vi "LV to ITX 2.2 2D w X&Y.vi"(0 "Commands":string, 1 "Kill X&Y waves?":bool=TRUE, 4 "Y Array name":string, 5 "filename":path, 6 "Y 1D Array":dbl[](array[numeric]), 7 "Notes":string, 8 "X  Array name":string, 9 "X 1D Array":dbl[](array[numeric]), 10 "2D Array name":string, 11 "2D Array":dbl[][](array[numeric])) -> (3 "file":path)   [LabVIEW 2016, in "LV to ITX.lvclass"]
uses:
  LV to ITX.lvclass
panel:
  out "Commands":string
  out "String":string
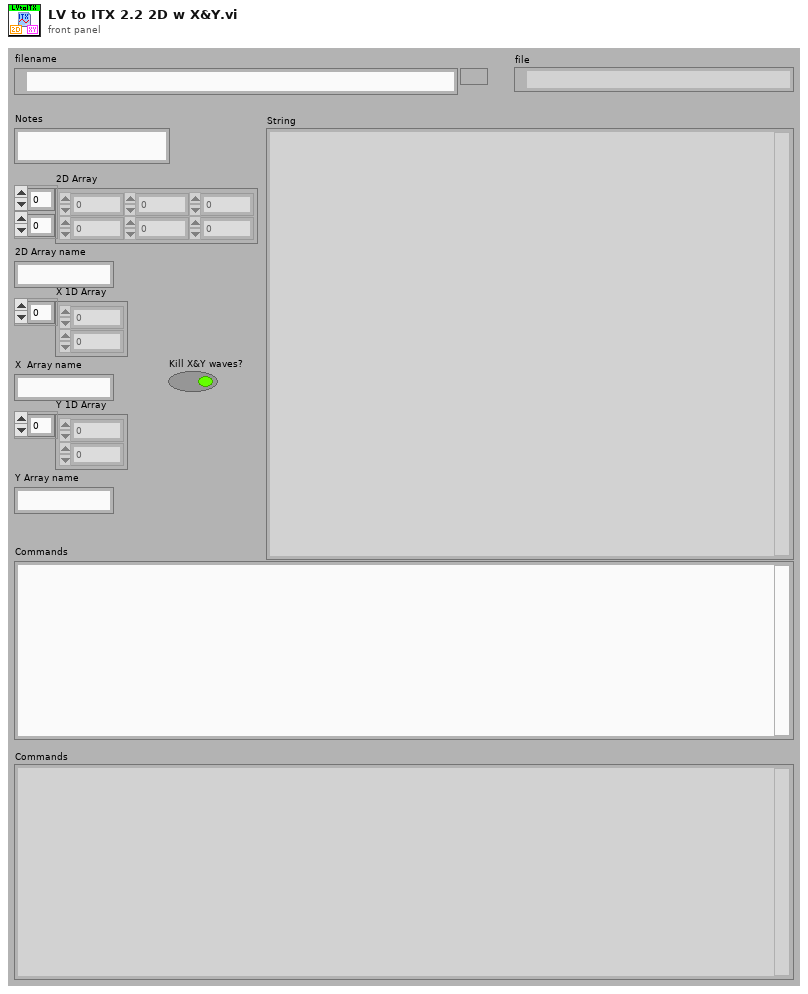
[diagram p1: front panel]
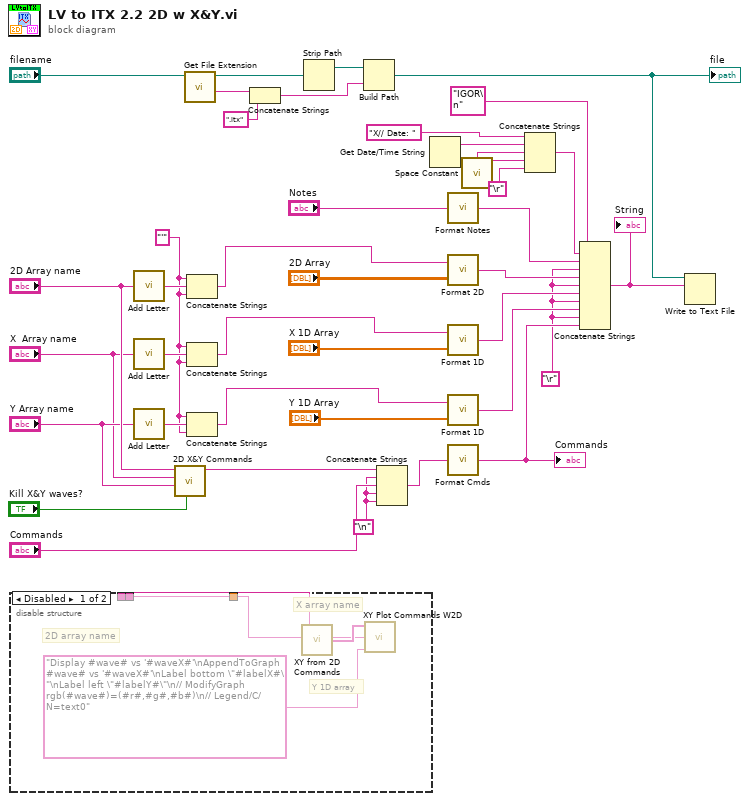
[diagram p0: block diagram]
diagram:
  w13 = "'" ("string")
  w2 = "\n"
  w27 = "\r"
  n1 = disable-structure shown="Disabled" {
    disable-tunnel: _ -> [w45 _]
    disable-tunnel: _ -> [w44 _]
    disable-tunnel: _ -> [w41 _]
    frame Disabled {
      # "Y 1D array"
      # "2D array name"
      # "X array name"
      n2 = call "XY from 2D Commands.vi"("Y 1D Array"=w44, "2D wave"=w45) -> ("wavenames"=w43:string[])
      n3 = call "XY Plot Commands W2D.vi"("wavenames"=w43, "input string"="Display #wave# vs '#waveX#'\nAppendToGraph #wave# vs '#waveX#'\nLabel bottom \"#labelX#\"\nLabel left \"#labelY#\"\n// ModifyGraph rgb(#wave#)=(#r#,#g#,#b#)\n// Legend/C/N=text0", "X wave"=w41) -> ()  [unwired: 2 in, 1 out]
    }
    frame Enabled {
    }
  }
  n4 = call "Add Letter.vi"("String"="2D Array name") -> ("output string"=w16:string)
  n5 = call "Add Letter.vi"("String"="X  Array name") -> ("output string"=w15:string)
  n6 = call "Add Letter.vi"("String"="Y Array name") -> ("output string"=w14:string)
  n7 = call "2D X&Y Commands.vi"("Kill X&Y waves?"="Kill X&Y waves?", "Y wave"="Y Array name", "X wave"="X  Array name", "2D wave"="2D Array name") -> ("result string"=w7:string)  [unwired: 6 in, 1 out]
  n8 = call <vilib>:"Get File Extension.vi"("file"="filename") -> ("filename without extension"=w23:string, "dup file"=w20:path)  [unwired: 1 in, 8 out]
  n9 = Concatenate Strings(w13, w16, w13) -> (w10:string)
  n10 = Concatenate Strings(w13, w15, w13) -> (w11:string)
  n11 = Concatenate Strings(w13, w14, w13) -> (w12:string)
  n12 = Concatenate Strings(w23, ".itx") -> (w18:string)
  n13 = Strip Path(path=w20) -> (stripped path=w19:path)  [unwired: 1 out]
  n14 = Build Path(base path=w19, name or relative path=w18) -> (appended path=w3:path)
  "file" <- w3
  n15 = Concatenate Strings(w7, w2, "Commands", w2, w2) -> (w21:string)
  n16 = Get Date/Time String() -> (date string=w38:string, time string=w39:string)  [unwired: 3 out]
  n17 = call "Format Notes.vi"("Notes"="Notes") -> ("String"=w28:string)
  n18 = call "Format 2D.vi"("2D Array"="2D Array", "2D Array name"=w10) -> ("String"=w32:string)
  n19 = call "Format 1D.vi"("X 1D Array"="X 1D Array", "X  Array name"=w11) -> ("String"=w31:string)
  n20 = call "Format 1D.vi"("X 1D Array"="Y 1D Array", "X  Array name"=w12) -> ("String"=w30:string)
  n21 = call "Format Cmds.vi"("Commands"=w21) -> ("String"=w29:string)
  "Commands" <- w29
  n22 = call <vilib>:"Space Constant.vi"() -> ("String"=w25:string)
  n23 = Concatenate Strings("X// Date: " ("format string"), w38, w25, w39, "\r") -> (w37:string)
  n24 = Concatenate Strings("IGOR\n", w37, w28, w27, w32, w27, w31, w27, w30, w27, w29) -> (w26:string)
  "String" <- w26
  n25 = Write to Text File(file (use dialog)=w3, text=w26) -> ()  [unwired: 1 in, 4 out]
